vi "Average.vi"(2 "averg #":dbl=0.95, 3 "Input":dbl, 4 "Previous\nValue":dbl) -> (1 "Output":dbl)   [LabVIEW 2012]
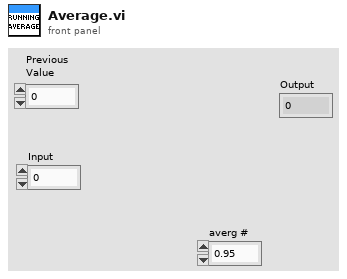
[diagram p1: front panel]
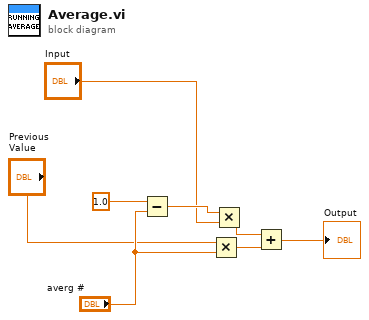
[diagram p0: block diagram]
diagram:
  n1 = Subtract(x=1.0, y="averg #") -> (x-y=w6:dbl)
  n2 = Multiply(x="Previous\nValue", y="averg #") -> (x*y=w8:dbl)
  n3 = Multiply(x=w6, y="Input") -> (x*y=w7:dbl)
  n4 = Add(x=w7, y=w8) -> (x+y=→"Output":dbl)
